vi "Initialize.vi"(7 "Error Query (False)":bool, 8 "error in (no error)":errorcluster, 9 "Reset (True)":bool=TRUE, 10 "ID Query (True)":bool, 11 "VISA resource name":refnum<visa-resource-name>="GPIB0::3::INSTR") -> (0 "error out":errorcluster, 3 "VISA resource name out":refnum<visa-resource-name>)   [LabVIEW 2018, in "Keithley 3706.lvlib"]
uses:
  <instrlib>/Keithley 3706/Keithley 3706.lvlib
panel:
  in  "Serial Configuration":T1={"Baud Rate"=9600, "Parity"=0, "Data Bits"=7, "Stop Bits"=10, "Flow Control"=0} {"Flow Control" items=["None", "XON/XOFF", "RTS/CTS", "XON/XOFF & RTS/CTS", "DTR/DSR", "XON/XOFF & DTR/DSR"]; "Stop Bits" items=["1.0"=10, "1.5"=15, "2.0"=20]; "Data Bits" items=["7"=7, "8"=8]; "Parity" items=["None", "Odd", "Even", "Mark", "Space"]; "Baud Rate" items=["300"=300, "600"=600, "1200"=1200, "2400"=2400, "4800"=4800, "9600"=9600, "19200"=19200]}
  # "(c) 2016 Keithley Instruments, Inc.  ALL RIGHTS RESERVED."
  # "Automatic"
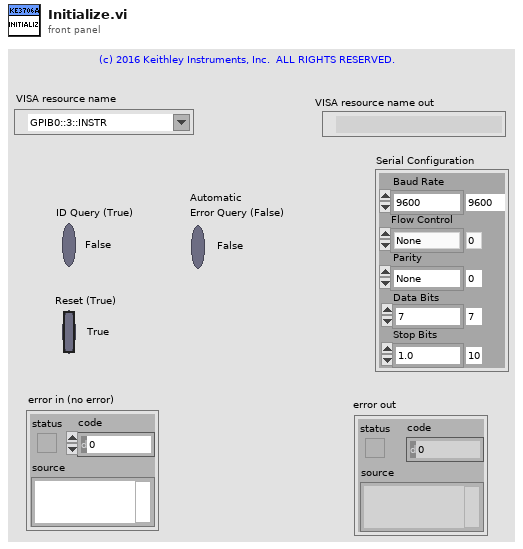
[diagram p1: front panel]
types:
  T1 = cluster{"Baud Rate":u32, "Parity":u16, "Data Bits":u16, "Stop Bits":u16, "Flow Control":u16}
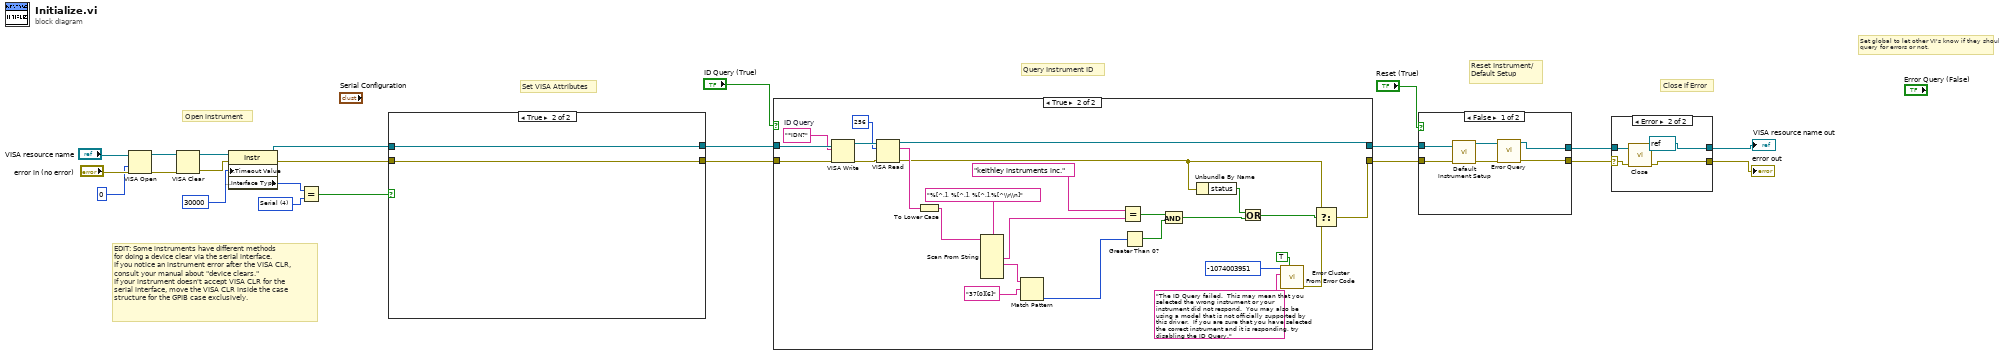
[diagram p0: block diagram]
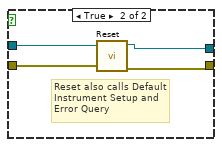
[diagram p3: hidden frame]
diagram:
  w15 = u16 4 items=["GPIB"=1, "VXI"=2, "GPIB-VXI"=3, "Serial"=4, "PXI"=5, "TCPIP"=6, "USB"=7] ("Interface Information:Interface Type")
  # "Set global to let other VI's know if they should\nquery for errors or not."
  # "Close if Error"
  # "Reset Instrument/\nDefault Setup"
  # "Query Instrument ID"
  # "Set VISA Attributes"
  # "Open instrument"
  # "EDIT: Some instruments have different methods\nfor doing a device clear via the serial interface.  \nIf you notice an instrument error after the VISA CLR,\nconsult your manual about \"device clears.\"  \nIf your instrument doesn't accept VISA CLR for the\nserial interface, move the VISA CLR inside the case \nstructure for the GPIB case exclusively."
  n1 = VISA Open(access mode=0, error in (no error)="error in (no error)", VISA resource name="VISA resource name") -> (VISA resource name=w21:refnum<visa-resource-name>, error out=w20:errorcluster)  [unwired: 2 in]
  n2 = VISA Clear(VISA resource name=w21, error in (no error)=w20) -> (VISA resource name out=w19:refnum<visa-resource-name>, error out=w18:errorcluster)
  n3 = property class="Instr"(reference=w19, error in=w18, "General Settings:Timeout Value"=30000) -> (reference out=w12:refnum<visa-resource-name>, error out=w13:errorcluster, "Interface Information:Interface Type"=w16:u16)
  n4 = Equal?(x=w16, y=w15) -> (x = y?=w14:bool)
  n5 = case shown="True" w14 {
    tunnel: w13 -> [w24 w26]
    tunnel: w12 -> [w25 w27]
    tunnel: [w25 w27] -> w10
    tunnel: [w24 w26] -> w9
    frame False {
      # "EDIT: Remove interfaces not\nsupported by your instrument."
      # "GPIB, TCP/IP, and USB Interface"
    }
    frame True {
    }
  }
  n6 = case shown="True" "ID Query (True)" {
    tunnel: w10 -> [w29 w55]
    tunnel: w9 -> [w28 w54]
    tunnel: [w29 w49] -> w7
    tunnel: [w28 w31] -> w6
    frame False {
    }
    frame True {
      w53 = "*IDN?"  # ID Query
      n7 = VISA Write(VISA resource name=w55, write buffer=w53, error in (no error)=w54) -> (VISA resource name out=w52:refnum<visa-resource-name>, error out=w51:errorcluster)  [unwired: 1 out]
      n8 = VISA Read(VISA resource name=w52, byte count=u32 256, error in (no error)=w51) -> (VISA resource name out=w49:refnum<visa-resource-name>, read buffer=w48:string, error out=w36:errorcluster)  [unwired: 1 out]
      n9 = To Lower Case(string=w48) -> (all lower case string=w47:string)
      n10 = Scan From String(format string="%[^,], %[^,], %[^,],%[^\\r\\n]", input string=w47) -> (output 1=w30:string, output 2=w44:string)  [unwired: 8 in, 3 out]
      n11 = Match Pattern(string=w44, regular expression="37[0][6]") -> (offset past match=w42:i32)  [unwired: 1 in, 3 out]
      n12 = Equal?(x="keithley instruments inc." ("regular expression"), y=w30) -> (x = y?=w41:bool)
      n13 = Greater Than 0?(x=w42) -> (x > 0?=w40:bool)
      n14 = And(x=w41, y=w40) -> (x .and. y?=w38:bool)
      n15 = Unbundle By Name(w36) -> ("status"=w39:bool)
      n16 = Or(x=w39, y=w38) -> (x .or. y?=w37:bool)
      n17 = call <vilib>:"Error Cluster From Error Code.vi"("show call chain? (False)"=TRUE, "error message (\"\")"="The ID Query failed.  This may mean that you selected the wrong instrument or your instrument did not respond.  You may also be using a model that is not officially supported by this driver.  If you are sure that you have selected the correct instrument and it is responding, try disabling the ID Query." ("Source (VI Name)"), "error code (0)"=-1074003951 ("Code")) -> ("error out"=w32:errorcluster)  [unwired: 6 in]
      n18 = Select(t=w36, s=w37, f=w32) -> (s? t:f=w31:errorcluster)
    }
  }
  n19 = case shown="False" "Reset (True)" {
    tunnel: w7 -> [w61 w65]
    tunnel: w6 -> [w60 w63]
    tunnel: [w57 w64] -> w4
    tunnel: [w56 w62] -> w5
    frame False {
      n20 = call <instrlib>:"Default Instrument Setup.vi"("error in (no error)"=w60, "VISA resource name"=w61) -> ("error out"=w58:errorcluster, "VISA resource name out"=w59:refnum<visa-resource-name>)  [unwired: 8 in]
      n21 = call <instrlib>:"Error Query.vi"("error in (no error)"=w58, "VISA resource name"=w59) -> ("error out"=w56:errorcluster, "VISA resource name output"=w57:refnum<visa-resource-name>)  [unwired: 6 in, 2 out]
    }
    frame True {
      # "Reset also calls Default Instrument Setup and Error Query"
      n22 = call <instrlib>:"Reset.vi"("error in (no error)"=w63, "VISA resource name"=w65) -> ("error out"=w62:errorcluster, "VISA resource name out"=w64:refnum<visa-resource-name>)  [unwired: 8 in]
    }
  }
  n23 = case shown="Error" w5 {
    selector: w5 -> [w66 w69]
    tunnel: w4 -> [w67 w70]
    tunnel: [w67 refnum<visa-resource-name> refnum ("VISA resource name out")] -> w3
    tunnel: [w66 w68] -> w2
    frame No Error {
    }
    frame Error {
      n24 = call <instrlib>:"Close.vi"("error in (no error)"=w69, "VISA resource name"=w70) -> ("error out"=w68:errorcluster)  [unwired: 9 in]
    }
  }
  "VISA resource name out" <- w3
  "error out" <- w2
